vi "Get TCP Link.vi"(8 "error in (no error)":errorcluster, 10 "IP Address":string, 11 "connection info in":T1) -> (0 "error out":errorcluster, 3 "connection info out":T1)   [LabVIEW 2016, in "Assert API Components.lvlib" / "Assert Service.lvlib" / "Assert Service.lvclass"]
uses:
  Assert Service.lvclass
  <vilib>/NI/STM/TCP/TCP Connection Info.ctl
  <vilib>/NI/STM/SubVIs/MetaDataElement.ctl
  <vilib>/NI/STM/TCP/Get Connection Reference (TCP).vi
  <vilib>/Utility/tcp.llb/UDP Multicast Read-Only Open.vi
  <vilib>/NI/STM/NI STM.lvlib
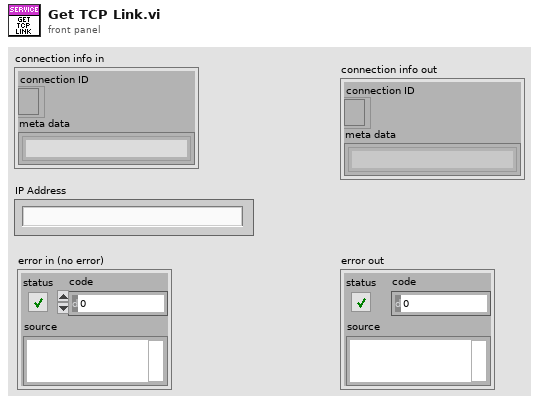
[diagram p1: front panel]
types:
  T1 = typedef "NI STM.lvlib/TCP Connection Info.ctl" = cluster{"connection ID":refnum<k5>, "meta data":T2[]}
  T2 = typedef "NI STM.lvlib/MetaDataElement.ctl" = string
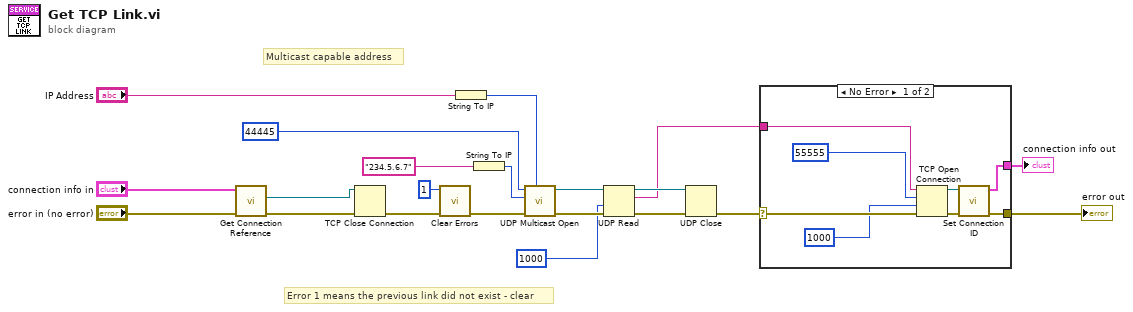
[diagram p0: block diagram]
diagram:
  # "Multicast capable address"
  # "Error 1 means the previous link did not exist - clear"
  n1 = call-poly <vilib>:"Get Connection Reference.vi"("error in"="error in (no error)", "connection info in"="connection info in") -> ("error out"=w18:errorcluster, "connection ID out"=w16:refnum<k5>)  [unwired: 8 out]
  n2 = TCP Close Connection(connection ID=w16, error in (no error)=w18) -> (error out=w15:errorcluster)  [unwired: 2 out]
  n3 = call <vilib>:"Clear Errors.vi"("error in (no error)"=w15, "specific error code to clear (0: all)"=1) -> ("error out"=w7:errorcluster)  [unwired: 4 in, 1 out]
  n4 = String To IP(1:"IP Address") -> (0:w2:u32)
  n5 = String To IP(1:"234.5.6.7" ("address")) -> (0:w4:u32)
  n6 = call-poly <vilib>:"UDP Multicast Open.vi"("net address"=w2, "error in (no error)"=w7, "multicast addr"=w4, "port"=u16 44445) -> ("error out"=w13:errorcluster, "connection ID"=w12:refnum<k16>)  [unwired: 5 in, 1 out]
  n7 = UDP Read(connection ID=w12, timeout ms (25000)=1000, 8:w13) -> (data out=w3:string, error out=w9:errorcluster, 3:w10:refnum<k16>)  [unwired: 1 in, 2 out]
  n8 = UDP Close(connection ID=w10, 8:w9) -> (error out=w8:errorcluster)  [unwired: 1 out]
  n9 = case shown="No Error" w8 {
    selector: w8 -> [w24 w29]
    tunnel: [w28 _] -> w21
    tunnel: [w25 w29] -> w20
    tunnel: w3 -> [w23 _]
    frame No Error {
      n10 = TCP Open Connection(address=w23, remote port or service name=u16 55555 ("remote port"), timeout ms (60000)=1000, error in (no error)=w24) -> (connection ID=w27:refnum<k5>, error out=w25:errorcluster)  [unwired: 1 out]
      n11 = call "Set Connection ID.vi"("TCP Network Connection in"=w27) -> ("connection info out"=w28:T1)  [unwired: 10 in]
    }
    frame Error {
    }
  }
  "connection info out" <- w21
  "error out" <- w20
